vi "Turning Movment.vi"(5 "Tolerance":dbl, 6 "Turn Time":dbl, 7 "Relative Angle":dbl, 8 "GyroDevRef":T1, 11 "RobotDriveDevRef":T4={"DevStatus"={"status"=FALSE, "code"=0, "source"=""}, "Motors[]"=[], "Square Inputs"=FALSE, "Max Output"=1.0, "Isochronous"=FALSE}) -> (2 "Finished?":bool)   [LabVIEW 2012]
uses:
  <vilib>/Rock Robotics/WPI/RobotDrive/WPI_RobotDriveDevRef.ctl
  <vilib>/Rock Robotics/WPI/MotorControl/WPI_MotorControlDeviceRef.ctl
  <vilib>/Rock Robotics/SystemInterfaces/Typedef/FPGA_TypedefDigitalModule.ctl
  <vilib>/Rock Robotics/SystemInterfaces/DIO/FPGA_DIOPWMChannel.ctl
  <vilib>/Rock Robotics/WPI/PWM/WPI_PWMDeadband.ctl
  <vilib>/Rock Robotics/WPI/CAN/Jaguar/SubVIs/WPI_CANJaguar_ControlMode.ctl
  <vilib>/Rock Robotics/WPI/PWM/WPI_PWMTransform_ConPane.ctl
  <vilib>/Rock Robotics/WPI/Gyro/WPI_GyroDevRef.ctl
  <vilib>/Rock Robotics/SystemInterfaces/Typedef/FPGA_TypedefAnalogModule.ctl
  <vilib>/Rock Robotics/SystemInterfaces/AI/FPGA_AIChannel.ctl
  <vilib>/addons/control/pid/pid.llb/PID (DBL).vi
  <vilib>/Rock Robotics/WPI/RobotDrive/WPI_RobotDriveArcadeDrive_Standard(NoSaturation).vi
  <vilib>/addons/control/pid/NI_PID_pid.lvlib
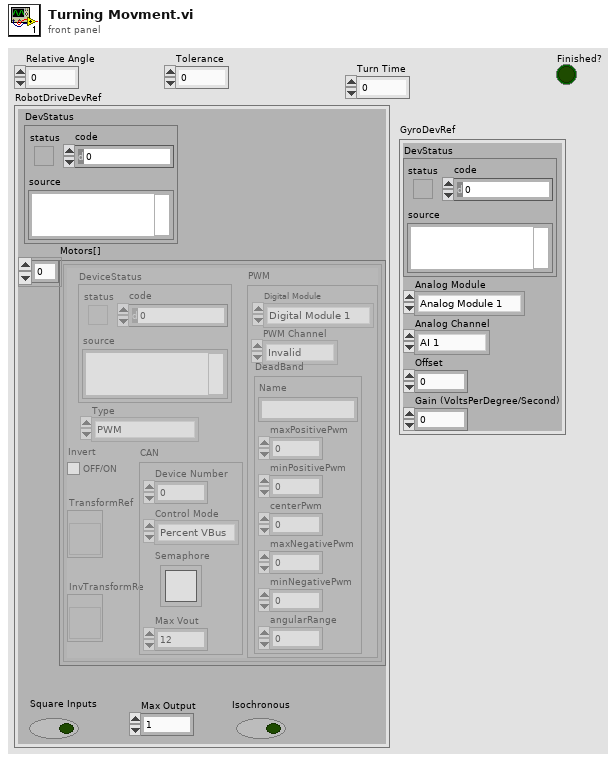
[diagram p1: front panel]
types:
  T1 = typedef "WPI_GyroDevRef.ctl" = cluster{"DevStatus":errorcluster, "Analog Module":T2, "Analog Channel":T3, "Offset":dbl, "Gain (VoltsPerDegree/Second)":dbl}
  T2 = typedef "FPGA_TypedefAnalogModule.ctl" = enum16{"Analog Module 1", "Analog Module 2"}
  T3 = typedef "FPGA_AIChannel.ctl" = enum8{"AI 1", "AI 2", "AI 3", "AI 4", "AI 5", "AI 6", "AI 7", "AI 8", "Invalid"}
  T4 = typedef "WPI_RobotDriveDevRef.ctl" = cluster{"DevStatus":errorcluster, "Motors[]":T5[], "Square Inputs":bool, "Max Output":dbl, "Isochronous":bool}
  T5 = typedef "WPI_MotorControlDeviceRef.ctl" = cluster{"DeviceStatus":errorcluster, "Type":enum16{"PWM", "CAN"}, "PWM":cluster{"Digital Module":T6, "PWM Channel":T7, "DeadBand":T8}, "CAN":cluster{"Device Number":u8, "Control Mode":T9, "Semaphore":T10, "Max Vout":dbl}, "Invert":bool, "TransformRef":T11, "InvTransformRef":T11}
  T6 = typedef "FPGA_TypedefDigitalModule.ctl" = enum16{"Digital Module 1", "Digital Module 2"}
  T7 = typedef "FPGA_DIOPWMChannel.ctl" = enum8{"PWM 1", "PWM 2", "PWM 3", "PWM 4", "PWM 5", "PWM 6", "PWM 7", "PWM 8", "PWM 9", "PWM 10", "Invalid"}
  T8 = typedef "WPI_PWMDeadband.ctl" = cluster{"Name":string, "maxPositivePwm":i32, "minPositivePwm":i32, "centerPwm":i32, "maxNegativePwm":i32, "minNegativePwm":i32, "angularRange":u16}
  T9 = typedef "WPI_CANJaguar_ControlMode.ctl" = enum8{"Percent VBus", "Current", "Speed", "Position", "Voltage"}
  T10 = typedef "Semaphore RefNum" = refnum<k1>
  T11 = typedef "WPI_PWMTransform_ConPane.ctl" = refnum<vi>
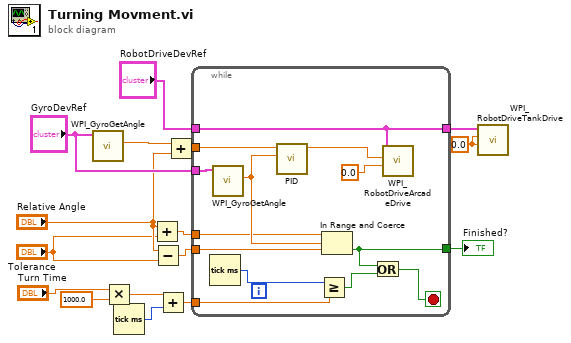
[diagram p0: block diagram]
diagram:
  w2 = 0.0 ("Left axis value")
  n1 = call <vilib>:"WPI_GyroGetAngle.vi"("GyroDevRef"="GyroDevRef") -> ("Angle"=w16:dbl)  [unwired: 7 in, 3 out]
  n2 = Multiply(x="Turn Time", y=1000.0) -> (x*y=w10:dbl)
  n3 = Tick Count (ms)() -> (millisecond timer value=w9:u32)
  n4 = Add(x="Relative Angle", y="Tolerance") -> (x+y=w5:dbl)
  n5 = Subtract(x="Relative Angle", y="Tolerance") -> (x-y=w4:dbl)
  n6 = Add(x=w10, y=w9) -> (x+y=w8:dbl)
  n7 = Add(x=w16, y="Relative Angle") -> (x+y=w15:dbl)
  n8 = while {
    tunnel: w15 -> [w29]
    tunnel: "RobotDriveDevRef" -> [w18]
    tunnel: "GyroDevRef" -> [w26]
    tunnel: w8 -> [w25]
    tunnel: w5 -> [w22]
    tunnel: w4 -> [w21]
    tunnel: [w18] -> w3
    tunnel: [w17] -> w1
    stop <- w19 stop-if-true
    n9 = Tick Count (ms)() -> (millisecond timer value=w24:u32)
    n10 = call <vilib>:"WPI_GyroGetAngle.vi"("GyroDevRef"=w26) -> ("Angle"=w23:dbl)  [unwired: 7 in, 3 out]
    n11 = call-poly <vilib>:"PID.vi"("process variable"=w23, "setpoint"=w29) -> ("output"=w27:dbl)  [unwired: 8 in, 1 out]
    n12 = Greater Or Equal?(x=w24, y=w25) -> (x >= y?=w20:bool)
    n13 = In Range and Coerce(upper limit=w22, x=w23, lower limit=w21) -> (In Range?=w17:bool)  [unwired: 1 out]
    n14 = Or(x=w17, y=w20) -> (x .or. y?=w19:bool)
    n15 = call-poly <vilib>:"WPI_RobotDriveArcadeDrive.vi"("Y axis value"=0.0, "X axis value"=w27, "RobotDriveDevRef"=w18) -> ()  [unwired: 6 in, 3 out]
  }
  "Finished?" <- w1
  n16 = call <vilib>:"WPI_RobotDriveTankDrive.vi"("Right axis value"=w2, "Left axis value"=w2, "RobotDriveDevRef"=w3) -> ()  [unwired: 6 in, 3 out]
